vi "setting.vi"() -> ()   [LabVIEW 2017]
panel:
  out "x与y？":bool
  out "x-y":dbl
  out "x+y":dbl
  out "范围内？ 3":bool
  out "数据 2":i32
  out "控件值:获取":variant
  in  "数据字符串":string
  out "子字符串 2":string
  out "数组":i32[](array[numeric])
  out "添加的数组 2":string[][](array[string])
  out "添加的数组":string[][](array[string])
  out "数据":string[][](array[string])
  in  "y 2":dbl[](array[numeric])
  in  "y":dbl[](array[numeric])
  in  "x":dbl[](array[numeric])
  out "XY图":cluster{"x":dbl[], "y 2":dbl[]}[](graph)
  out "保存名":string
  out "数据保存路径":path
  out "时间字符串":string
  out "数字 3":i32
  out "数字 2":i32
  out "数字":dbl
  out "子字符串":string
  out "匹配偏移量":i32
  out "匹配+剩余字符串":string
  in  "字符串":string
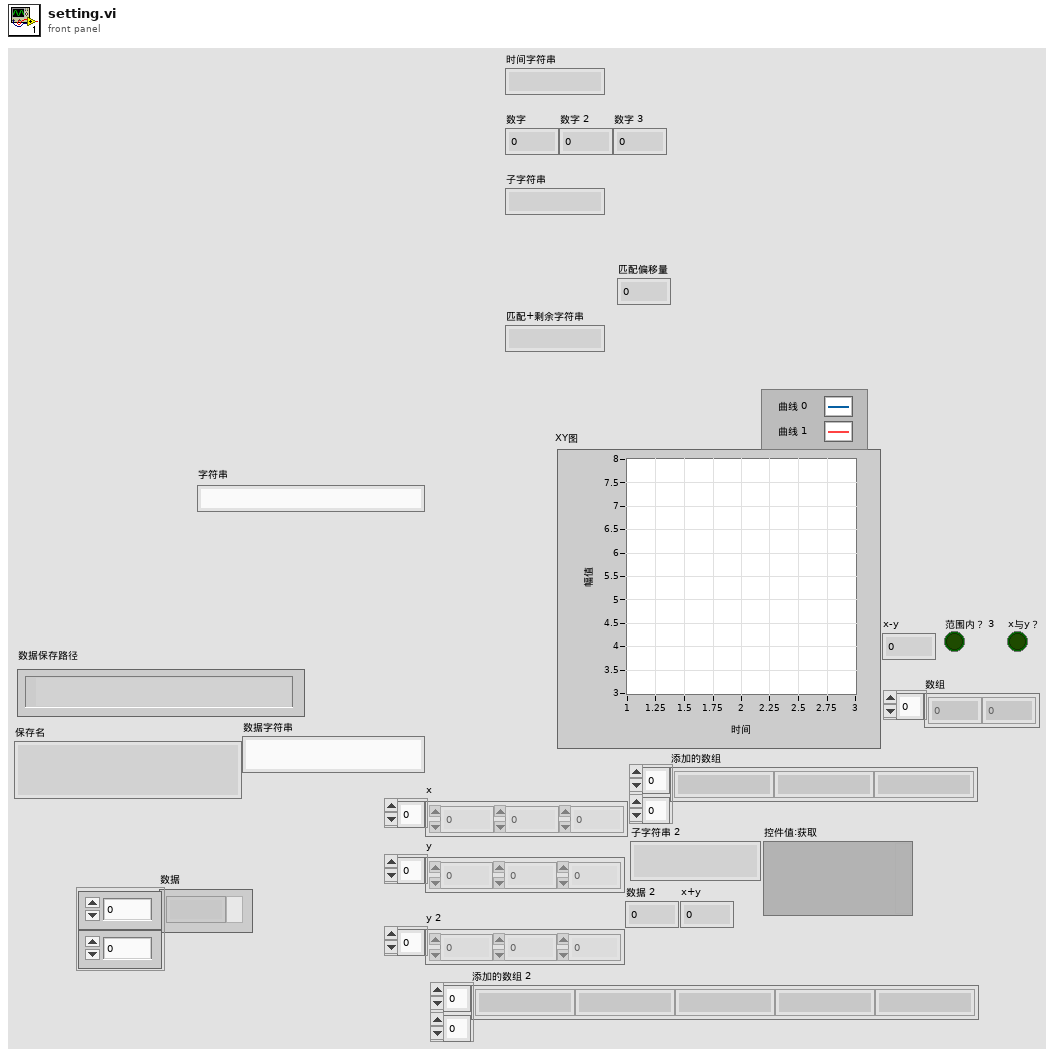
[diagram p1: front panel]
types:
  T1 = enum16{"open", "open or create", "create or replace", "create", "open (read-only)"}
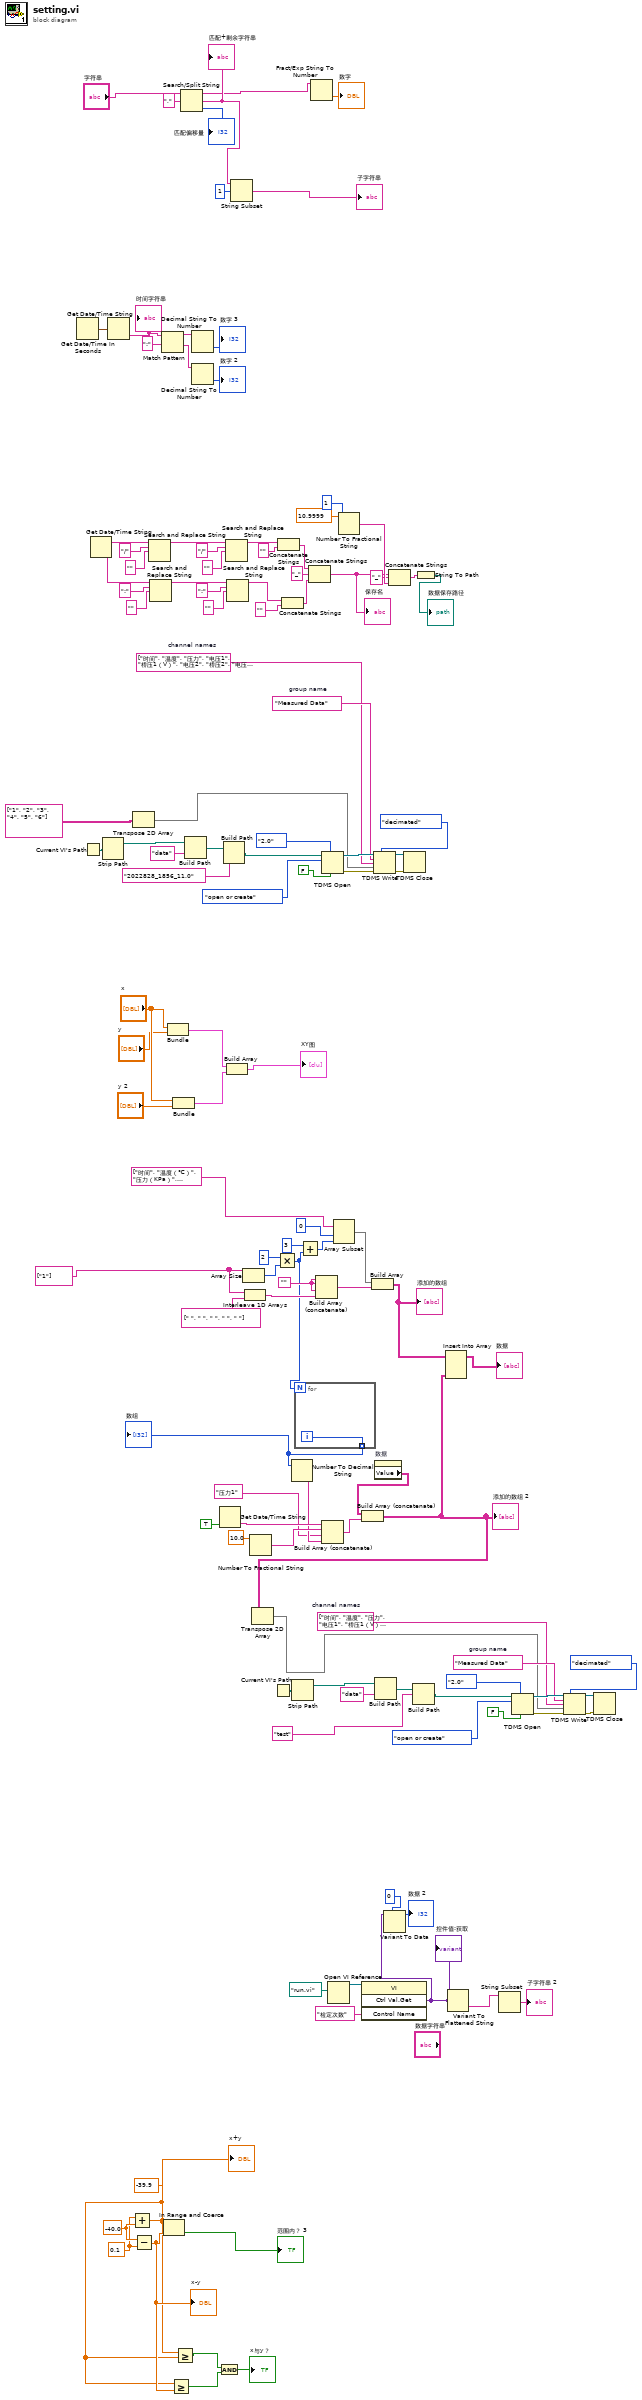
[diagram p0: block diagram]
diagram:
  w1 = -39.9 ("x")
  w8 = 0.1
  w9 = -40.0
  w23 = "Measured Data"  # group name
  w22 = string[] ["时间", "温度", "压力", "电压1", "桥压1（V）", "电压2", "桥压2", "电压3", "桥压3", "电压4", "桥压4", "电压5", "桥压5"]  # channel names
  w38 = string[] ["1"]
  w52 = ""
  w69 = "Measured Data"  # group name
  w68 = string[] ["时间", "温度", "压力", "电压1", "桥压1（V）", "电压2", "桥压2", "电压3", "桥压3", "电压4", "桥压4", "电压5", "桥压5"]  # channel names
  n1 = Get Date/Time In Seconds() -> (seconds since 1Jan1904=w116:timestamp)
  n2 = Current VI's Path() -> (path=w80:path)
  n3 = Get Date/Time String() -> (date string=w100:string, time string=w88:string)  [unwired: 3 in]
  n4 = Strip Path(path=w80) -> (stripped path=w79:path)  [unwired: 1 out]
  n5 = Get Date/Time String(seconds (now)=w116) -> (time string=w112:string)  [unwired: 2 in, 1 out]
  "时间字符串" <- w112
  n6 = Add(x=w8, y=w9) -> (x+y=w2:dbl)
  "x+y" <- w2
  n7 = Transpose 2D Array(2D array=string[][] [["1", "2", "3"], ["4", "5", "6"]]) -> (transposed array=w75:string[][])
  n8 = Subtract(x=w9, y=w8) -> (x-y=w6:dbl)
  "x-y" <- w6
  n9 = Search and Replace String(input string=w100, search string="/" ("搜索字符串"), replace string="" ("替换字符串(\"\")")) -> (result string=w107:string)  [unwired: 5 in, 3 out]
  n10 = Search and Replace String(input string=w88, search string=":" ("搜索字符串"), replace string="" ("替换字符串(\"\")")) -> (result string=w94:string)  [unwired: 5 in, 3 out]
  n11 = Match Pattern(string=w112, regular expression=":" ("正则表达式")) -> (before substring=w115:string, after substring=w114:string)  [unwired: 1 in, 2 out]
  n12 = In Range and Coerce(upper limit=w2, x=w1, lower limit=w6) -> (In Range?=→"范围内？ 3":bool)  [unwired: 1 out]
  n13 = Bundle("x"="x", "y"="y") -> (w62:cluster{"x":dbl[], "y":dbl[]})  [unwired: 1 in]
  n14 = Greater Or Equal?(x=w1, y=w6) -> (x >= y?=w5:bool)
  n15 = Bundle("x"="x", "y 2"="y 2") -> (w61:cluster{"x":dbl[], "y 2":dbl[]})  [unwired: 1 in]
  n16 = Greater Or Equal?(x=w2, y=w1) -> (x >= y?=w3:bool)
  n17 = Search/Split String(string="字符串", search string/char (-)="," ("搜索字符串/字符(-)")) -> (substring before match=w118:string, match + rest of string=w121:string, offset of match=→"匹配偏移量":i32)  [unwired: 1 in]
  "匹配+剩余字符串" <- w121
  n18 = Build Path(base path=w79, name or relative path="data" ("字符串")) -> (appended path=w78:path)
  n19 = Decimal String To Number(string=w115) -> (number=→"数字 3":i32)  [unwired: 2 in, 1 out]
  n20 = Decimal String To Number(string=w114) -> (number=→"数字 2":i32)  [unwired: 2 in, 1 out]
  n21 = Get Date/Time String(want seconds? (F)=TRUE ("disable buffering (T)")) -> (time string=w47:string)  [unwired: 2 in, 1 out]
  n22 = And(x=w3, y=w5) -> (x .and. y?=→"x与y？":bool)
  n23 = Build Path(base path=w78, name or relative path="2022828_1856_11.0" ("名称或相对路径")) -> (appended path=w83:path)
  n24 = Search and Replace String(input string=w107, search string="/" ("搜索字符串"), replace string="" ("替换字符串(\"\")")) -> (result string=w104:string)  [unwired: 5 in, 3 out]
  n25 = Build Array(w62, w61) -> (→"XY图":cluster{"x":dbl[], "y 2":dbl[]}[])
  n26 = Search and Replace String(input string=w94, search string=":" ("搜索字符串"), replace string="" ("替换字符串(\"\")")) -> (result string=w90:string)  [unwired: 5 in, 3 out]
  n27 = String Subset(string=w121, offset (0)=1 ("偏移量(0)")) -> (substring=→"子字符串":string)  [unwired: 1 in]
  n28 = Array Size(array=w38) -> (size(s)=w59:i32)
  n29 = Interleave 1D Arrays(w38, string[] [" ", " ", " ", " ", " "]) -> (w53:string[])
  n30 = Number To Fractional String(number=10.0 ("数字")) -> (F-format string=w46:string)  [unwired: 3 in]
  n31 = Current VI's Path() -> (path=w33:path)
  n32 = Multiply(x=2, y=w59) -> (x*y=w44:i32)
  n33 = Concatenate Strings(w104, "" ("字符串")) -> (w102:string)
  n34 = Concatenate Strings(w90, "" ("字符串")) -> (w87:string)
  n35 = Strip Path(path=w33) -> (stripped path=w32:path)  [unwired: 1 out]
  n36 = for {
    N: w44 -> [_]
    tunnel: [w125] -> w42 mode=indexing
    i -> [w125]
  }
  "数组" <- w42
  n37 = Number To Decimal String(number=w42) -> (decimal integer string=w41:string[])  [unwired: 1 in]
  n38 = Add(x=3, y=w44) -> (x+y=w55:i32)
  n39 = Concatenate Strings(w102, "_" ("字符串"), w87) -> (w84:string)
  "保存名" <- w84
  n40 = Fract/Exp String To Number(string=w118) -> (number=→"数字":dbl)  [unwired: 3 in, 1 out]
  n41 = Build Array (concatenate)(w52, w52, w52, w53) -> (w50:string[])
  n42 = TDMS Open(6:FALSE ("disable buffering (T)"), 7:enum16{"1.0", "2.0"}."2.0" ("file format version (2.0)"), 10:T1."open or create" ("operation"), 11:w83) -> (0:w81:errorcluster, 3:w77:refnum<k34>)  [unwired: 3 in]
  n43 = Build Array (concatenate)(w47, w46, "压力1", w41) -> (w45:string[])
  n44 = Open VI Reference(vi path=path "run.vi" ("VI路径")) -> (vi reference=w16:refnum<vi>)  [unwired: 5 in, 1 out]
  n45 = Array Subset(array=string[] ["时间", "温度（℃）", "压力（KPa）", "电压1（V）", "桥压1（V）", "电压2（V）", "桥压2（V）", "电压3（V）", "桥压3（V）", "电压4（V）", "桥压4（V）", "电压5（V）", "桥压5（V）"], index=0 ("索引"), length=w55) -> (w51:string[])
  n46 = Number To Fractional String(number=10.9999 ("数字"), precision (6)=i16 1 ("精度(6)")) -> (F-format string=w86:string)  [unwired: 2 in]
  n47 = invoke class="VI" method="Ctrl Val.Get"(reference=w16, "Control Name"="检定次数" ("控件名")) -> ("Get Control Value Variant"=w12:variant)  [unwired: 2 in, 3 out]
  "控件值:获取" <- w12
  n48 = Build Array(w51, w50) -> (w39:string[][])
  "添加的数组" <- w39
  n49 = TDMS Write(0:w77, 1:enum16{"decimated", "interleaved"}."decimated" ("数据布局（0:降采样）"), 5:w69, 7:w68, 9:w75, 11:w81) -> (4:w76:refnum<k34>, 15:w82:errorcluster)  [unwired: 2 out]
  n50 = property on="数据" class="Arr (严格)"() -> ("Value"=w43:string[][])  [unwired: 2 in, 2 out]
  n51 = Build Array (concatenate)(w43, w45) -> (w19:string[][])
  "添加的数组 2" <- w19
  n52 = Transpose 2D Array(2D array=w19) -> (transposed array=w18:string[][])
  n53 = Build Path(base path=w32, name or relative path="data" ("字符串")) -> (appended path=w31:path)
  n54 = Variant To Data(type=0, Variant=w12) -> (data=→"数据 2":i32)  [unwired: 1 in, 1 out]
  n55 = Concatenate Strings(w84, "_" ("字符串"), w86) -> (w101:string)
  n56 = TDMS Close(8:w82, 11:w76) -> ()  [unwired: 2 out]
  n57 = Build Path(base path=w31, name or relative path="test") -> (appended path=w36:path)
  n58 = String To Path(string=w101) -> (path=→"数据保存路径":path)
  n59 = Insert Into Array(array=w39, new element=w19) -> (→"数据":string[][])  [unwired: 2 in]
  n60 = Variant To Flattened String(Variant=w12) -> (data string=w14:string)  [unwired: 1 out]
  n61 = String Subset(string=w14) -> (substring=→"子字符串 2":string)  [unwired: 2 in]
  n62 = TDMS Open(6:FALSE ("disable buffering (T)"), 7:enum16{"1.0", "2.0"}."2.0" ("file format version (2.0)"), 10:T1."open or create" ("operation"), 11:w36) -> (0:w34:errorcluster, 3:w30:refnum<k34>)  [unwired: 3 in]
  n63 = TDMS Write(0:w30, 1:enum16{"decimated", "interleaved"}."decimated" ("数据布局（0:降采样）"), 5:w23, 7:w22, 9:w18, 11:w34) -> (4:w29:refnum<k34>, 15:w35:errorcluster)  [unwired: 2 out]
  n64 = TDMS Close(8:w35, 11:w29) -> ()  [unwired: 2 out]
